vi "build_etc_command_map.vi"() -> (0 "excite_controls_xt600":map{string, string}(c390)={"AssignLedToGroup"="lg=", "ClearAlarm"="ca", "Connect"="co\r", "Disconnect"="dc\r", "DosimeterInformation"="do?", "EnableGroup"="ge=", "GetDateLED"="md?", "GetFullWidthHalfMaximumValueLED"="lf?", "GetGeneratorPulseMode"="pm?", "GetHighSpeedModeSettingLED"="hs?", "GetIntensity"="ip?", "GetLedGroupMembers"="lgx?", "GetLedHours"="lh?\r", "GetLedOffStates"="of?", "GetLedOnStates"="on?", "GetLedSequencing"="ts?", "GetLogicTTL"="tl?", "GetMaximumTemperaturesLED"="mt?", "GetMinimumPulseWidthLED"="mw?", "GetMinimumtemperaturesLED"="nt?", "GetModePWM"="sc?", "GetNameLED"="ln?", "GetScreenBrightness"="lb?", "GetScreenSaverTimeout"="st?", "GetSerialNumber"="ls?", "GetSignalDelayTime"="dt?", "GetSignalOffTime"="ft?", "GetSignalOnTime"="ot?", "GetSoftwareVersion"="sv?\r", "GetSpeakerVolume"="vo?", "GetTemperature"="gt?", "GetTemperatureHysteresisLED"="th?", "GetTimeoutTTL"="ti?", "GetTriggerAdvanceTime"="tt?", "GetTypeLED"="lt?", "GetUnitSerialNumber"="sn?", "GetUnitStatus"="us?\\r", "GetUnitsPWM"="su?", "GetWaveLengthLED"="lw?", "IsGroupEnabled"="ge?", "IsOneAnalogSetting"="oa?", "IsTerminalMode"="tm?", "LockFrontPanel"="lo", "MinimumIntensityPercentage"="ni?", "SaveSettings"="sa", "ScreenLCD"="ss?", "SerialType"="si?", "SetGeneratorPulseMode"="pm=", "SetHighSpeedIntensityLED"="CY", "SetHighSpeedModeLED"="hs=", "SetIntensity"="ip=", "SetLedSequencing"="ts=", "SetLogicTTL"="tl=", "SetModePWM"="sc=x", "SetOneAnalogSetting"="oa=", "SetScreenBrightness"="lb=", "SetScreenSaverTimeout"="st=", "SetSignalDelayTime"="dt=", "SetSignalOffTime"="ft=", "SetSignalOnTime"="ot=", "SetSpeakerVolume"="vo=", "SetStatesLED"="8Y", "SetTerminalMode"="nt?", "SetTriggerAdvanceTime"="tt=", "SetUnitsPWM"="su=", "StartPWM"="is=1", "StatusPWM"="is", "StopPWM"="is=0", "TurnAllLedOff"="of=a", "TurnAllLedOn"="on=", "TurnLedOff"="of=", "TurnLedOn"="on=w,x,y,z", "UnlockFrontPanel"="ul", "WavelengthRange"="wr?"}, 1 "xcite_commands_xled1":map{string, string}(c390)={"ClearAlarm"="ca", "Connect"="co", "Disconnect"="dc", "GetDateLED"="md?", "GetFullWidthHalfMaximumValueLED"="lf?", "GetGeneratorPulseMode"="pm?", "GetHighSpeedModeSettingLED"="hs?", "GetIntensity"="ip?", "GetLedHours"="lh?", "GetLedOffStates"="of?", "GetLedOnStates"="on?", "GetMaximumTemperaturesLED"="mt?", "GetMinimumPulseWidthLED"="mw?", "GetMinimumtemperaturesLED"="nt?", "GetModePWM"="sc?", "GetNameLED"="ln?", "GetScreenBrightness"="lb?", "GetScreenSaverTimeout"="st?", "GetSerialNumber"="ls?", "GetSignalDelayTime"="dt?", "GetSignalOffTime"="ft?", "GetSignalOnTime"="ot?", "GetSoftwareVersion"="sv?", "GetSpeakerVolume"="vo?", "GetTemperature"="gt?", "GetTemperatureHysteresisLED"="th?", "GetTriggerAdvanceTime"="tt?", "GetTypeLED"="lt?", "GetUnitSerialNumber"="sn?", "GetUnitStatus"="us?", "GetUnitsPWM"="su?", "GetWaveLengthLED"="lw?", "LockFrontPanel"="lo", "ScreenLCD"="ss?", "SetGeneratorPulseMode"="mp=x", "SetHighSpeedIntensityLED"="CY", "SetHighSpeedModeLED"="hs=w,x,y,z", "SetIntensity"="ip=wwww,xxxx,yyyy,zzzz", "SetModePWM"="sc=x", "SetScreenBrightness"="lb=xxx", "SetScreenSaverTimeout"="st=xxxxx", "SetSignalDelayTime"="dt=wwwww,xxxxx,yyyyy,zzzzz", "SetSignalOffTime"="ft=wwwww,xxxxx,yyyyy,zzzzz", "SetSignalOnTime"="ot=wwwww,xxxxx,yyyyy,zzzzz", "SetSpeakerVolume"="vo=xxx", "SetStatesLED"="8Y", "SetTriggerAdvanceTime"="tt=wwwww,xxxxx,yyyyy,zzzzz", "SetUnitsPWM"="su=w,x,y,z", "StartPWM"="is=1", "StatusPWM"="is", "StopPWM"="is=0", "TurnAllLedOff"="of=a", "TurnAllLedOn"="on=a", "TurnLedOff"="of=w,x,y,z", "TurnLedOn"="on=w,x,y,z", "UnlockFrontPanel"="ul"}, 2 "xcite_commands_ex":map{string, string}(c390)={"DecrementIris"="--", "DisableShutterControl"="yy", "EnableExtendedCommands"="jj", "EnableShutterControl"="cc", "GetIntensity"="dd", "GetOutputPower"="pp", "GetPowerFactor"="??", "GetSerialNumber"="GSN", "GetTemperature"="gt", "IncrementIris"="++", "MinimumIntensityPercentage"="ni", "SetIntensity"="d", "SetOutputPower"="p"}, 3 "xcite_commands":map{string, string}(c390)={"ClearAlarm"="aa", "CloseShutter"="zz", "Connect"="tt", "GetIntensityH4"="ii", "GetLampHours"="hh", "GetSoftwareVersion"="vv", "GetUnitStatus"="uu", "LockFrontPanel"="ll", "OpenShutter"="mm", "SetIntensityH4"="i", "TurnLampOff"="ss", "TurnLampOn"="bb", "UnlockFrontPanel"="nn"}, 4 "xcite_controls_XT900":map{string, string}(c390)={"AssignLedToGroup"="lg=", "ClearAlarm"="ca", "Connect"="co", "Disconnect"="dc", "EnableGroup"="ge=", "GetDateLED"="md?", "GetFilterHD"="hd?", "GetFullWidthHalfMaximumValueLED"="lf?", "GetGainSetting"="ga?", "GetGeneratorPulseMode"="pm?", "GetHighSpeedModeSettingLED"="hs?", "GetIntensity"="ip?", "GetLedGroupMembers"="lgx?", "GetLedHours"="lh?", "GetLedOffStates"="of?", "GetLedOnStates"="on?", "GetLedSequencing"="ts?", "GetLogicTTL"="tl?", "GetMaximumTemperaturesLED"="mt?", "GetMinimumPulseWidthLED"="mw?", "GetMinimumtemperaturesLED"="nt?", "GetModePWM"="sc?", "GetNameLED"="ln?", "GetOpticalIntensitySensorADC"="re?", "GetPulseMode"="lc?", "GetScreenBrightness"="lb?", "GetScreenSaverTimeout"="st?", "GetSerialNumber"="ls?", "GetSignalDelayTime"="dt?", "GetSignalOffTime"="ft?", "GetSignalOnTime"="ot?", "GetSoftwareVersion"="sv?", "GetSpeakerVolume"="vo?", "GetTemperature"="gt?", "GetTemperatureHysteresisLED"="th?", "GetTimeoutTTL"="ti?", "GetTriggerAdvanceTime"="tt?", "GetTypeLED"="lt?", "GetUnitSerialNumber"="sn?", "GetUnitStatus"="us?", "GetUnitsPWM"="su?", "GetVirtualPower"="vp?", "GetWaveLengthLED"="lw?", "IsGroupEnabled"="ge?", "IsOneAnalogSetting"="oa?", "LockFrontPanel"="lo", "MinimumIntensityPercentage"="ni?", "SaveSettings"="sa", "ScreenLCD"="ss?", "SerialType"="si?", "SetFilterHD"="hd=", "SetGainSetting"="ga=", "SetGeneratorPulseMode"="pm=", "SetHighSpeedIntensityLED"="CY", "SetHighSpeedModeLED"="hs=", "SetIntensity"="ip=", "SetLedSequencing"="ts=", "SetLogicTTL"="tl=", "SetModePWM"="sc=", "SetOneAnalogSetting"="oa=", "SetPulseMode"="lc=", "SetScreenBrightness"="lb=", "SetScreenSaverTimeout"="st=", "SetSignalDelayTime"="dt=", "SetSignalOffTime"="ft=", "SetSignalOnTime"="ot=", "SetSpeakerVolume"="vo=", "SetStatesLED"="8Y", "SetTriggerAdvanceTime"="tt=", "SetUnitsPWM"="su=", "SetVirtualPower"="vp=", "StartPWM"="is=1", "StatusPWM"="is", "StopPWM"="is=0", "TurnAllLedOff"="of=a", "TurnAllLedOn"="on=a", "TurnLedOff"="of=", "TurnLedOn"="on=", "UnlockFrontPanel"="ul", "WavelengthRange"="wr?"})   [LabVIEW 2019, in "XCite.lvlib"]
doc: "VI to build maps for XCite commands. Outputs map readable command text to ACII commands that the XCite devices accept."
uses:
  XCite.lvlib
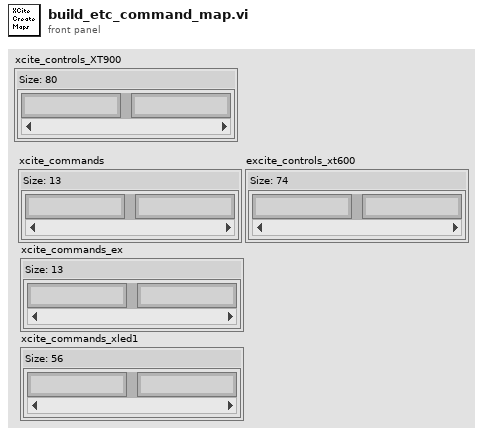
[diagram p1: front panel]
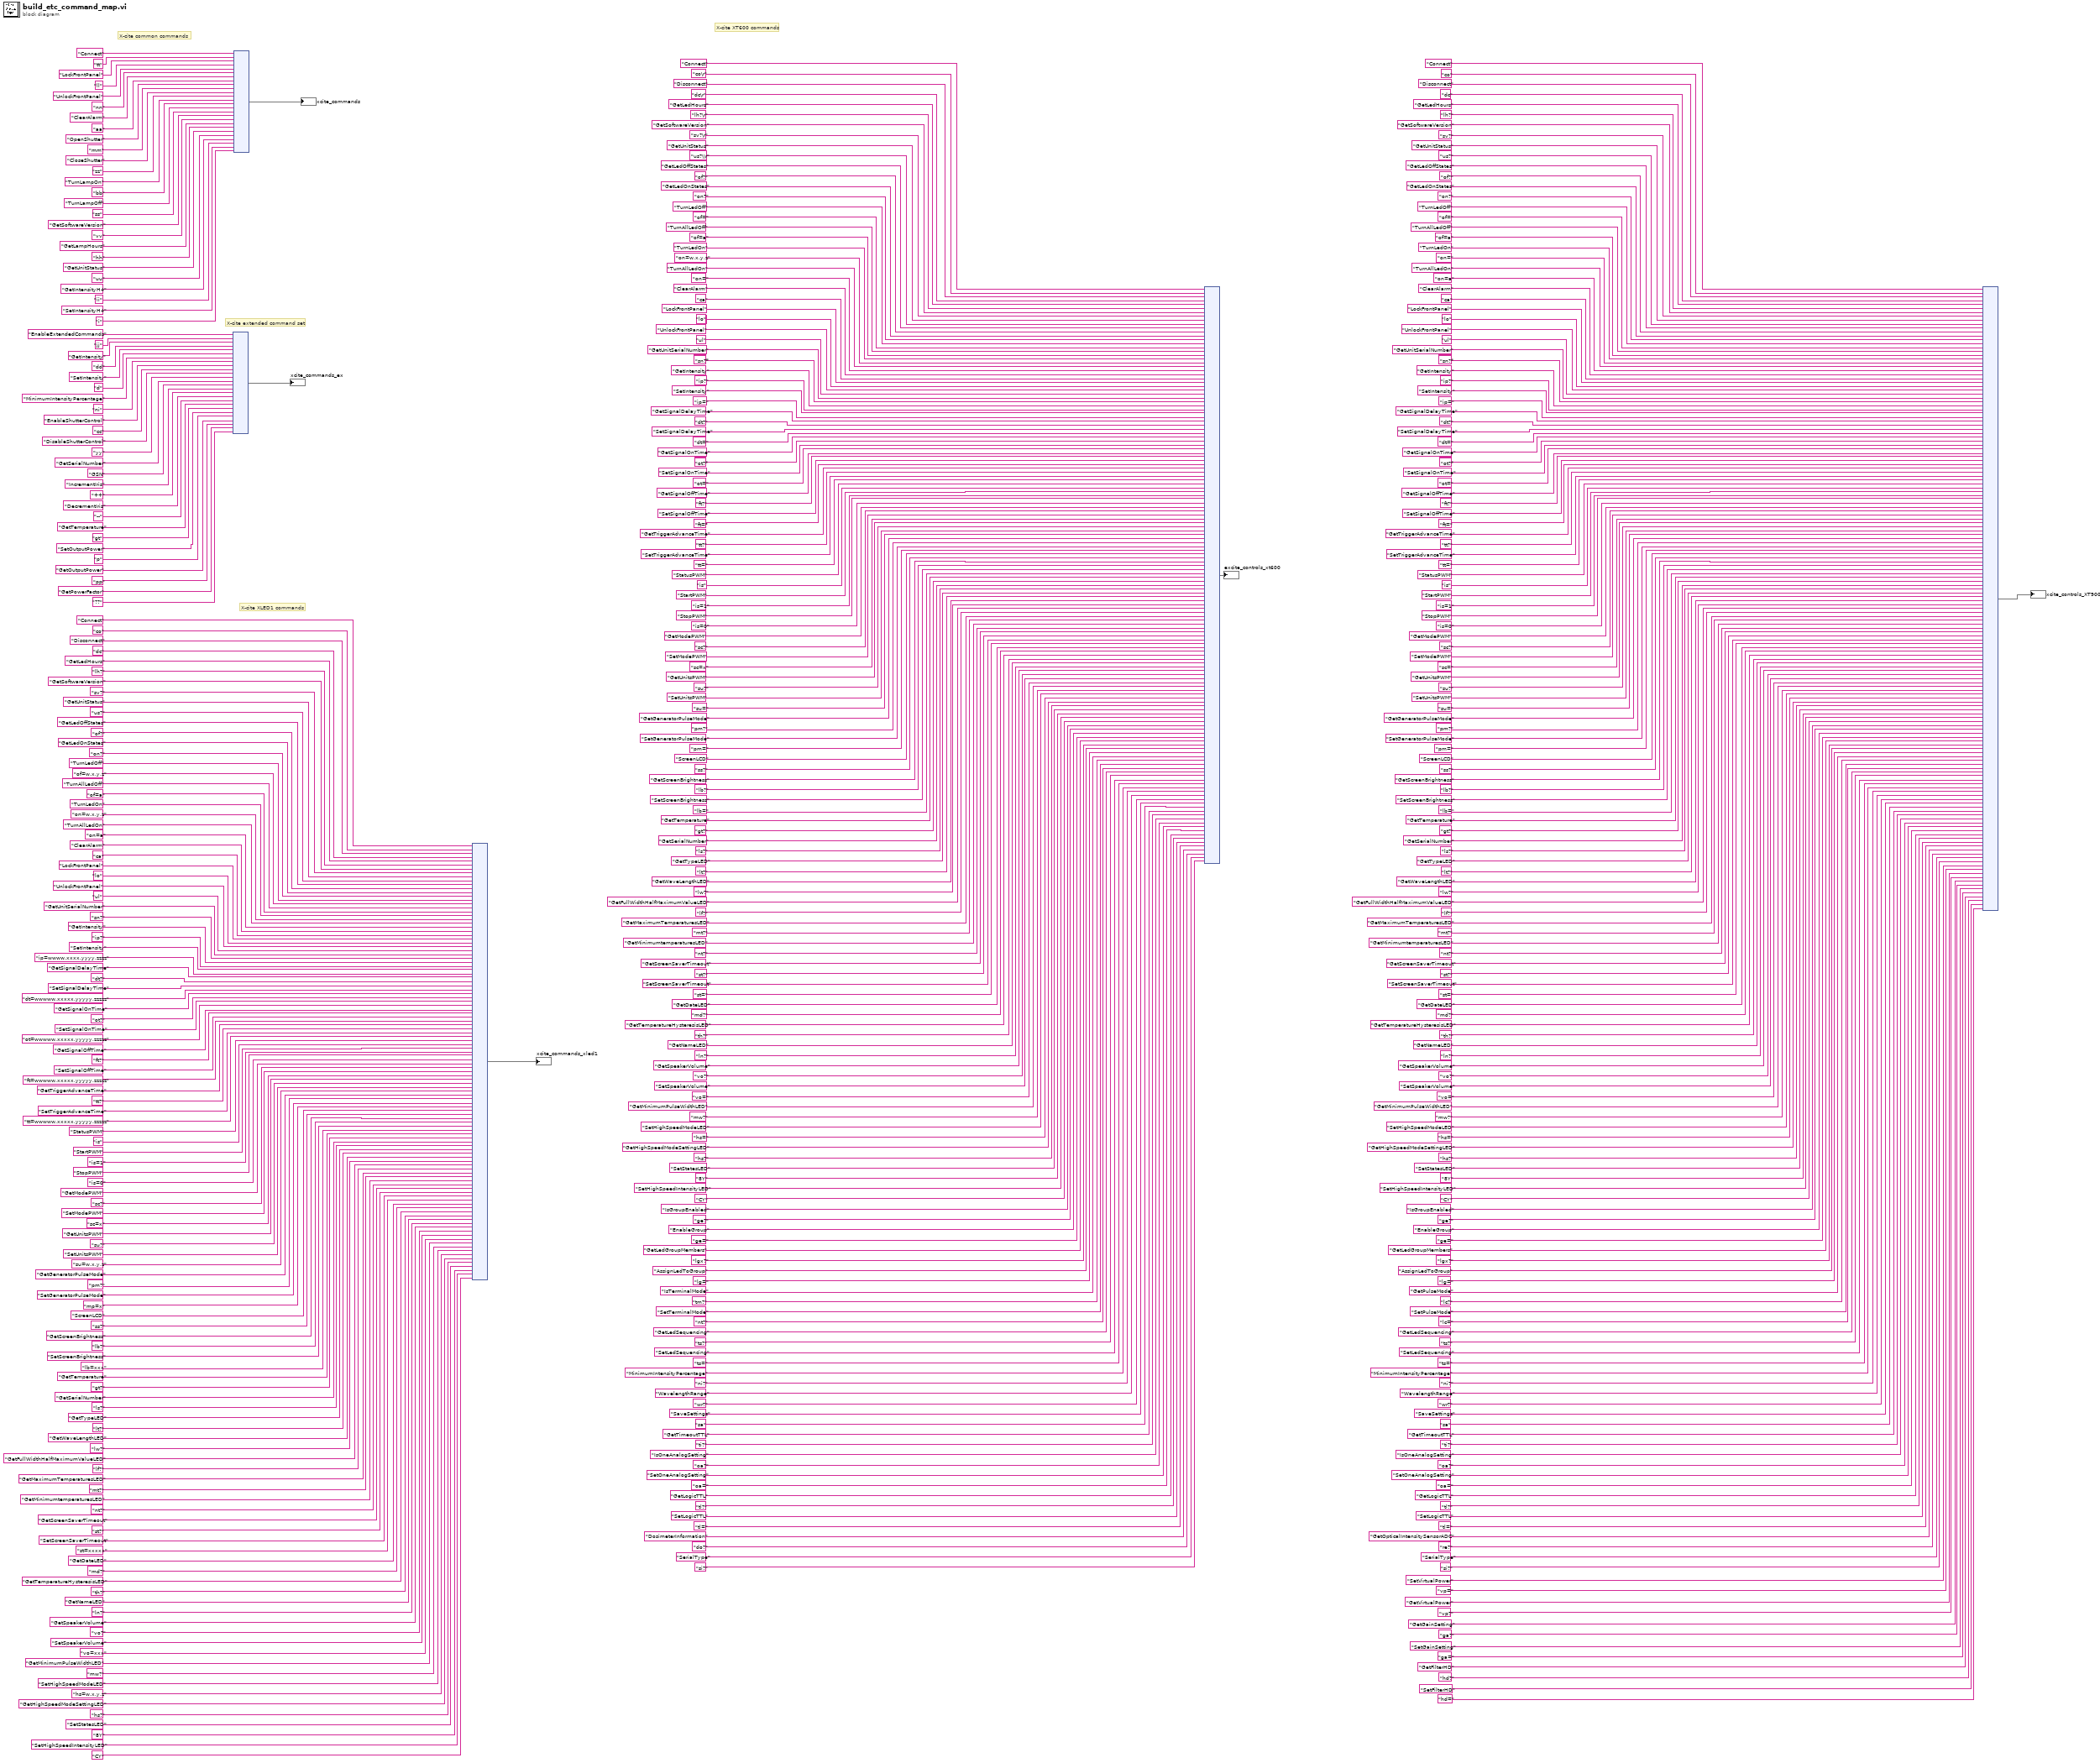
[diagram p0: block diagram]
diagram:
  (unwired) "ot?"
  (unwired) "sn?"
  (unwired) "lo"
  (unwired) "ot?"
  (unwired) "sn?"
  (unwired) "lo"
  # "X-cite XT600 commands"
  # "X-cite XLED1 commands"
  # "X-cite extended command set"
  # "X-cite common commands"
  n1 = node("EnableExtendedCommands", "jj", "GetIntensity", "dd", "SetIntensity", "d", "MinimumIntensityPercentage", "ni", "EnableShutterControl", "cc", "DisableShutterControl", "yy", "GetSerialNumber", "GSN", "IncrementIris", "++", "DecrementIris", "--", "GetTemperature", "gt", "SetOutputPower", "p", "GetOutputPower", "pp", "GetPowerFactor", "??") -> (→"xcite_commands_ex":map{string, string})
  n2 = node("Connect", "tt", "LockFrontPanel", "ll", "UnlockFrontPanel", "nn", "ClearAlarm", "aa", "OpenShutter", "mm", "CloseShutter", "zz", "TurnLampOn", "bb", "TurnLampOff", "ss", "GetSoftwareVersion", "vv", "GetLampHours", "hh", "GetUnitStatus", "uu", "GetIntensityH4", "ii", "SetIntensityH4", "i") -> (→"xcite_commands":map{string, string})
  n3 = node("Connect", "co", "Disconnect", "dc", "GetLedHours", "lh?", "GetSoftwareVersion", "sv?", "GetUnitStatus", "us?", "GetLedOffStates", "of?", "GetLedOnStates", "on?", "TurnLedOff", "of=w,x,y,z", "TurnAllLedOff", "of=a", "TurnLedOn", "on=w,x,y,z", "TurnAllLedOn", "on=a", "ClearAlarm", "ca", "LockFrontPanel", "lo", "UnlockFrontPanel", "ul", "GetUnitSerialNumber", "sn?", "GetIntensity", "ip?", "SetIntensity", "ip=wwww,xxxx,yyyy,zzzz", "GetSignalDelayTime", "dt?", "SetSignalDelayTime", "dt=wwwww,xxxxx,yyyyy,zzzzz", "GetSignalOnTime", "ot?", "SetSignalOnTime", "ot=wwwww,xxxxx,yyyyy,zzzzz", "GetSignalOffTime", "ft?", "SetSignalOffTime", "ft=wwwww,xxxxx,yyyyy,zzzzz", "GetTriggerAdvanceTime", "tt?", "SetTriggerAdvanceTime", "tt=wwwww,xxxxx,yyyyy,zzzzz", "StatusPWM", "is", "StartPWM", "is=1", "StopPWM", "is=0", "GetModePWM", "sc?", "SetModePWM", "sc=x", "GetUnitsPWM", "su?", "SetUnitsPWM", "su=w,x,y,z", "GetGeneratorPulseMode", "pm?", "SetGeneratorPulseMode", "mp=x", "ScreenLCD", "ss?", "GetScreenBrightness", "lb?", "SetScreenBrightness", "lb=xxx", "GetTemperature", "gt?", "GetSerialNumber", "ls?", "GetTypeLED", "lt?", "GetWaveLengthLED", "lw?", "GetFullWidthHalfMaximumValueLED", "lf?", "GetMaximumTemperaturesLED", "mt?", "GetMinimumtemperaturesLED", "nt?", "GetScreenSaverTimeout", "st?", "SetScreenSaverTimeout", "st=xxxxx", "GetDateLED", "md?", "GetTemperatureHysteresisLED", "th?", "GetNameLED", "ln?", "GetSpeakerVolume", "vo?", "SetSpeakerVolume", "vo=xxx", "GetMinimumPulseWidthLED", "mw?", "SetHighSpeedModeLED", "hs=w,x,y,z", "GetHighSpeedModeSettingLED", "hs?", "SetStatesLED", "8Y", "SetHighSpeedIntensityLED", "CY") -> (→"xcite_commands_xled1":map{string, string})
  n4 = node("Connect", "co\r", "Disconnect", "dc\r", "GetLedHours", "lh?\r", "GetSoftwareVersion", "sv?\r", "GetUnitStatus", "us?\\r", "GetLedOffStates", "of?", "GetLedOnStates", "on?", "TurnLedOff", "of=", "TurnAllLedOff", "of=a", "TurnLedOn", "on=w,x,y,z", "TurnAllLedOn", "on=", "ClearAlarm", "ca", "LockFrontPanel", "lo", "UnlockFrontPanel", "ul", "GetUnitSerialNumber", "sn?", "GetIntensity", "ip?", "SetIntensity", "ip=", "GetSignalDelayTime", "dt?", "SetSignalDelayTime", "dt=", "GetSignalOnTime", "ot?", "SetSignalOnTime", "ot=", "GetSignalOffTime", "ft?", "SetSignalOffTime", "ft=", "GetTriggerAdvanceTime", "tt?", "SetTriggerAdvanceTime", "tt=", "StatusPWM", "is", "StartPWM", "is=1", "StopPWM", "is=0", "GetModePWM", "sc?", "SetModePWM", "sc=x", "GetUnitsPWM", "su?", "SetUnitsPWM", "su=", "GetGeneratorPulseMode", "pm?", "SetGeneratorPulseMode", "pm=", "ScreenLCD", "ss?", "GetScreenBrightness", "lb?", "SetScreenBrightness", "lb=", "GetTemperature", "gt?", "GetSerialNumber", "ls?", "GetTypeLED", "lt?", "GetWaveLengthLED", "lw?", "GetFullWidthHalfMaximumValueLED", "lf?", "GetMaximumTemperaturesLED", "mt?", "GetMinimumtemperaturesLED", "nt?", "GetScreenSaverTimeout", "st?", "SetScreenSaverTimeout", "st=", "GetDateLED", "md?", "GetTemperatureHysteresisLED", "th?", "GetNameLED", "ln?", "GetSpeakerVolume", "vo?", "SetSpeakerVolume", "vo=", "GetMinimumPulseWidthLED", "mw?", "SetHighSpeedModeLED", "hs=", "GetHighSpeedModeSettingLED", "hs?", "SetStatesLED", "8Y", "SetHighSpeedIntensityLED", "CY", "IsGroupEnabled", "ge?", "EnableGroup", "ge=", "GetLedGroupMembers", "lgx?", "AssignLedToGroup", "lg=", "IsTerminalMode", "tm?", "SetTerminalMode", "nt?", "GetLedSequencing", "ts?", "SetLedSequencing", "ts=", "MinimumIntensityPercentage", "ni?", "WavelengthRange", "wr?", "SaveSettings", "sa", "GetTimeoutTTL", "ti?", "IsOneAnalogSetting", "oa?", "SetOneAnalogSetting", "oa=", "GetLogicTTL", "tl?", "SetLogicTTL", "tl=", "DosimeterInformation", "do?", "SerialType", "si?") -> (→"excite_controls_xt600":map{string, string})
  n5 = node("Connect", "co", "Disconnect", "dc", "GetLedHours", "lh?", "GetSoftwareVersion", "sv?", "GetUnitStatus", "us?", "GetLedOffStates", "of?", "GetLedOnStates", "on?", "TurnLedOff", "of=", "TurnAllLedOff", "of=a", "TurnLedOn", "on=", "TurnAllLedOn", "on=a", "ClearAlarm", "ca", "LockFrontPanel", "lo", "UnlockFrontPanel", "ul", "GetUnitSerialNumber", "sn?", "GetIntensity", "ip?", "SetIntensity", "ip=", "GetSignalDelayTime", "dt?", "SetSignalDelayTime", "dt=", "GetSignalOnTime", "ot?", "SetSignalOnTime", "ot=", "GetSignalOffTime", "ft?", "SetSignalOffTime", "ft=", "GetTriggerAdvanceTime", "tt?", "SetTriggerAdvanceTime", "tt=", "StatusPWM", "is", "StartPWM", "is=1", "StopPWM", "is=0", "GetModePWM", "sc?", "SetModePWM", "sc=", "GetUnitsPWM", "su?", "SetUnitsPWM", "su=", "GetGeneratorPulseMode", "pm?", "SetGeneratorPulseMode", "pm=", "ScreenLCD", "ss?", "GetScreenBrightness", "lb?", "SetScreenBrightness", "lb=", "GetTemperature", "gt?", "GetSerialNumber", "ls?", "GetTypeLED", "lt?", "GetWaveLengthLED", "lw?", "GetFullWidthHalfMaximumValueLED", "lf?", "GetMaximumTemperaturesLED", "mt?", "GetMinimumtemperaturesLED", "nt?", "GetScreenSaverTimeout", "st?", "SetScreenSaverTimeout", "st=", "GetDateLED", "md?", "GetTemperatureHysteresisLED", "th?", "GetNameLED", "ln?", "GetSpeakerVolume", "vo?", "SetSpeakerVolume", "vo=", "GetMinimumPulseWidthLED", "mw?", "SetHighSpeedModeLED", "hs=", "GetHighSpeedModeSettingLED", "hs?", "SetStatesLED", "8Y", "SetHighSpeedIntensityLED", "CY", "IsGroupEnabled", "ge?", "EnableGroup", "ge=", "GetLedGroupMembers", "lgx?", "AssignLedToGroup", "lg=", "GetPulseMode", "lc?", "SetPulseMode", "lc=", "GetLedSequencing", "ts?", "SetLedSequencing", "ts=", "MinimumIntensityPercentage", "ni?", "WavelengthRange", "wr?", "SaveSettings", "sa", "GetTimeoutTTL", "ti?", "IsOneAnalogSetting", "oa?", "SetOneAnalogSetting", "oa=", "GetLogicTTL", "tl?", "SetLogicTTL", "tl=", "GetOpticalIntensitySensorADC", "re?", "SerialType", "si?", "SetVirtualPower", "vp=", "GetVirtualPower", "vp?", "GetGainSetting", "ga?", "SetGainSetting", "ga=", "GetFilterHD", "hd?", "SetFilterHD", "hd=") -> (→"xcite_controls_XT900":map{string, string})
